vi "Get BufferLossless.vi"(11 "AI Current DAQmx Cont CFG in":refnum<class "AI Current DAQmx Cont CFG.lvclass">) -> (2 "BufferLossless":refnum<class "BufferLossless.lvclass">, 3 "AI Current DAQmx Cont CFG out":refnum<class "AI Current DAQmx Cont CFG.lvclass">)   [LabVIEW 2024, in "AI Current DAQmx Cont CFG.lvclass"]
uses:
  AI Current DAQmx Cont CFG.lvclass
  AI Current DAQmx Cont CFG.lvclass/AI Current DAQmx Cont CFG.ctl
  Buffers/BufferLossless/BufferLossless.lvclass
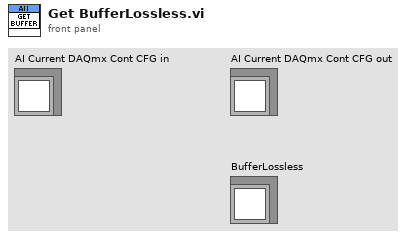
[diagram p1: front panel]
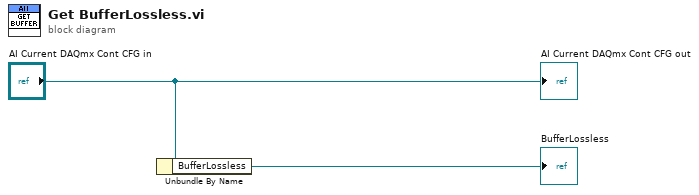
[diagram p0: block diagram]
diagram:
  n1 = Unbundle By Name("AI Current DAQmx Cont CFG in") -> ("BufferLossless"=→"BufferLossless":refnum<class "BufferLossless.lvclass">)
  "AI Current DAQmx Cont CFG out" <- "AI Current DAQmx Cont CFG in"
